vi "ServerTimestampName.vi"() -> (1 "message name":string)   [LabVIEW 2017, in "ServerComm.lvlib"]
doc: "Returns the following message name: ServerComm.ServerTimestamp. This message instructs NI InsightCM Server to return its current date and time as a timestamp. Use the ReceiveServerTimestamp to parse the server response."
uses:
  <vilib>/addons/InsightCM/Devices/Shared/Common/ServerComm/ServerComm.lvlib
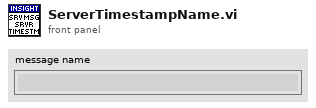
[diagram p1: front panel]
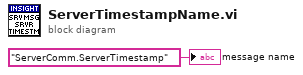
[diagram p0: block diagram]
diagram:
  "message name" <- "ServerComm.ServerTimestamp" ("ProcessName")
